vi "DB Path.vi"() -> (3 "DB Path":path)   [LabVIEW 2020, in "Settings.lvlib"]
uses:
  Settings.lvlib
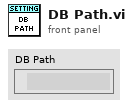
[diagram p1: front panel]
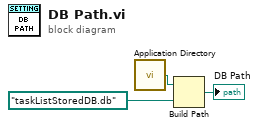
[diagram p0: block diagram]
diagram:
  n1 = call <vilib>:"Application Directory.vi"() -> ("Application Directory"=w3:path)
  n2 = Build Path(base path=w3, name or relative path=path "taskListStoredDB.db") -> (appended path=→"DB Path":path)
